vi "Blend Colors.vi"(1 "Target":u32(colorbox)=16448250, 2 "Source":u32(colorbox)) -> (0 "Array":u32[](array[numeric]))   [LabVIEW 2023, in "Freetype Drawer.lvlib"]
uses:
  Freetype Drawer.lvlib
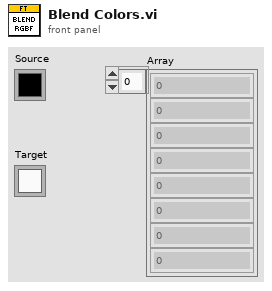
[diagram p1: front panel]
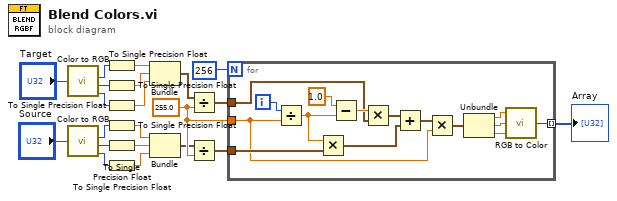
[diagram p0: block diagram]
diagram:
  w6 = sgl 255.0
  n1 = call <vilib>:"Color to RGB.vi"("Color"="Target") -> ("R"=w13:u8, "G"=w14:u8, "B"=w15:u8)  [unwired: 1 out]
  n2 = call <vilib>:"Color to RGB.vi"("Color"="Source") -> ("R"=w18:u8, "G"=w17:u8, "B"=w16:u8)  [unwired: 1 out]
  n3 = To Single Precision Float(number=w13) -> (single precision float=w7:sgl)
  n4 = To Single Precision Float(number=w14) -> (single precision float=w8:sgl)
  n5 = To Single Precision Float(number=w15) -> (single precision float=w9:sgl)
  n6 = To Single Precision Float(number=w18) -> (single precision float=w10:sgl)
  n7 = To Single Precision Float(number=w17) -> (single precision float=w12:sgl)
  n8 = To Single Precision Float(number=w16) -> (single precision float=w11:sgl)
  n9 = Bundle(w7, w8, w9) -> (w1:cluster{sgl, sgl, sgl})  [unwired: 1 in]
  n10 = Bundle(w10, w12, w11) -> (w2:cluster{sgl, sgl, sgl})  [unwired: 1 in]
  n11 = Divide(x=w1, y=w6) -> (x/y=w3:cluster{sgl, sgl, sgl})
  n12 = Divide(x=w2, y=w6) -> (x/y=w4:cluster{sgl, sgl, sgl})
  n13 = for {
    N: 256 -> [_]
    tunnel: [w24] -> w21 mode=indexing
    tunnel: w4 -> [w33]
    tunnel: w3 -> [w31]
    tunnel: w6 -> [w22]
    i -> [w36]
    n14 = Divide(x=w36, y=w22) -> (x/y=w35:sgl)
    n15 = Multiply(x=w35, y=w33) -> (x*y=w29:cluster{sgl, sgl, sgl})
    n16 = Subtract(x=sgl 1.0, y=w35) -> (x-y=w32:sgl)
    n17 = Multiply(x=w32, y=w31) -> (x*y=w30:cluster{sgl, sgl, sgl})
    n18 = Add(x=w30, y=w29) -> (x+y=w28:cluster{sgl, sgl, sgl})
    n19 = Multiply(x=w28, y=w22) -> (x*y=w23:cluster{sgl, sgl, sgl})
    n20 = Unbundle(w23) -> (w27:sgl, w26:sgl, w25:sgl)
    n21 = call <vilib>:"RGB to Color.vi"("B"=w25, "G"=w26, "R"=w27) -> ("Color"=w24:u32)
  }
  "Array" <- w21
